vi "Read Oil Presence.vi"(0 "Session Handle in":T1, 11 "error in (no error)":errorcluster) -> (4 "Session Handle out":T1, 6 "Present?":bool, 15 "error out":errorcluster)   [LabVIEW 2015, in "Gas.lvclass"]
uses:
  Gas.lvclass
  Typedefs/Session Handle.ctl
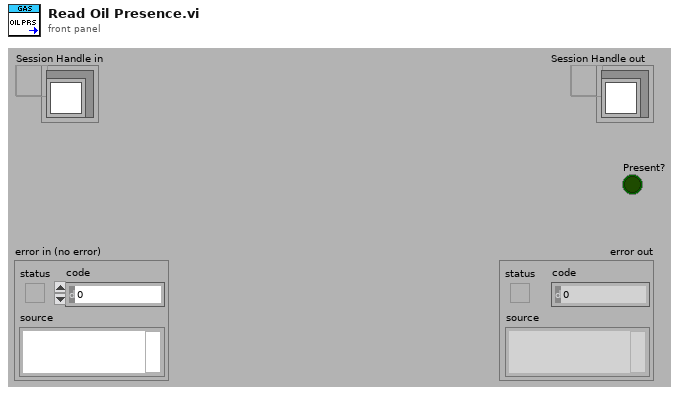
[diagram p1: front panel]
types:
  T1 = typedef "Gas.lvclass/Session Handle.ctl" = refnum<data-value>
  T2 = typedef "XNET Frame CAN.ctl" = cluster{"timestamp":timestamp, "payload":u8[], "identifier":u32, "type":T3, "extended?":bool, "echo?":bool}
  T3 = typedef "XNET Frame Type CAN.ctl" = u8
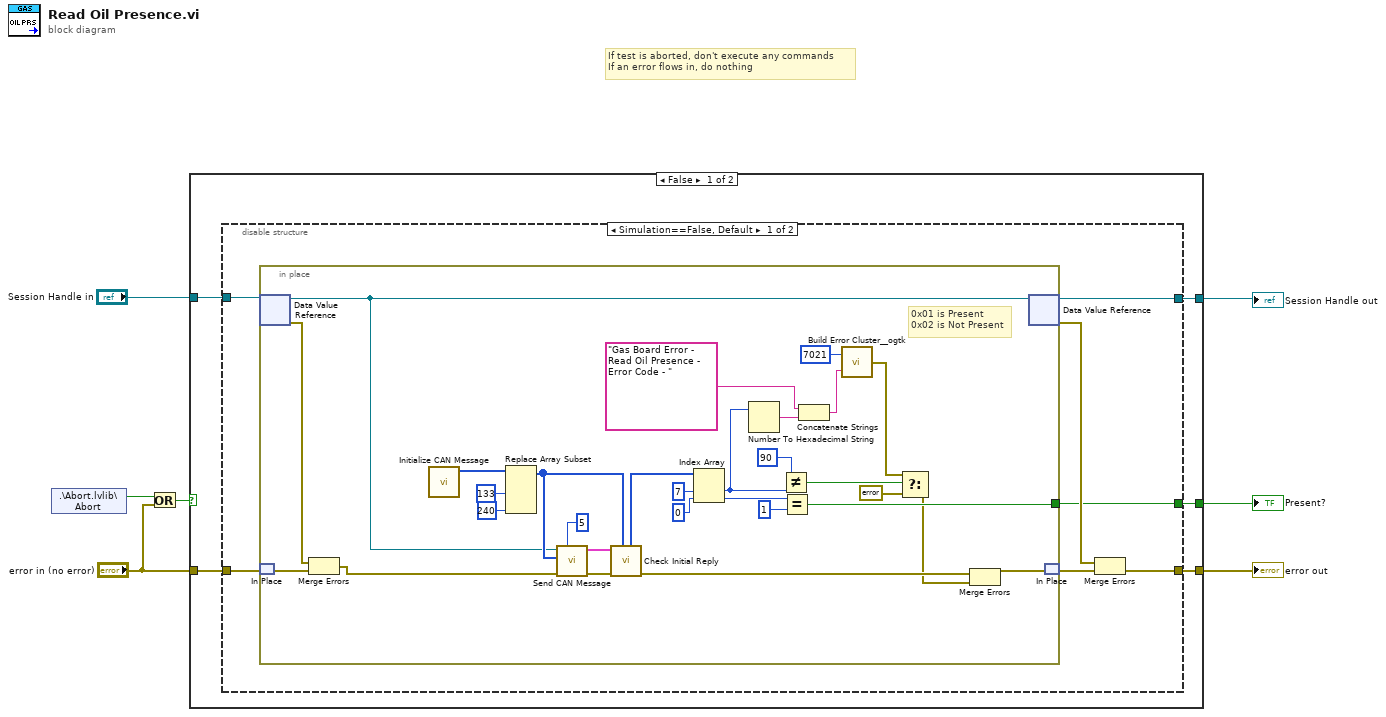
[diagram p0: block diagram]
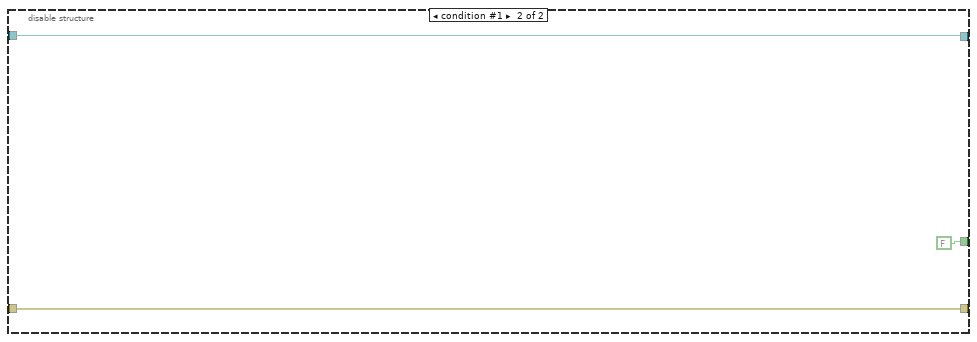
[diagram p2: hidden frame]
diagram:
  # "If test is aborted, don't execute any commands\nIf an error flows in, do nothing"
  n1 = shared-variable ".\\Abort.lvlib\\Abort"() -> (w4:bool)  [unwired: 1 in, 1 out]
  n2 = Or(x=w4, y="error in (no error)") -> (x .or. y?=w2:bool)
  n3 = case shown="False" w2 {
    tunnel: [w12 w53] -> w6
    tunnel: [w11 w52] -> w5
    tunnel: "Session Handle in" -> [w10 w53]
    tunnel: "error in (no error)" -> [w9 w52]
    tunnel: [w8 _] -> w1
    frame False {
      n4 = disable-structure shown="Simulation==False, Default" {
        disable-tunnel: [w19 w51] -> w12
        disable-tunnel: [w16 w50] -> w11
        disable-tunnel: w10 -> [w15 w51]
        disable-tunnel: w9 -> [w14 w50]
        disable-tunnel: [w13 FALSE] -> w8
        frame condition #0 (active) {
          n5 = in-place {
            in-place-border: [w31] -> w13
            # "0x01 is Present\n0x02 is Not Present"
            n6 = in-place-dvr #1(w15) -> (w25:refnum<class "Gas.lvclass">, w44:errorcluster)
            n7 = in-place-match #2(w14) -> (w43:errorcluster)
            n8 = Merge Errors(w44, w43) -> (w24:errorcluster)
            n9 = call "Initialize CAN Message.vi"() -> ("Initial Payload"=w45:u8[])  [unwired: 11 in]
            n10 = Replace Array Subset(array=w45, new element #1=u8 133 ("new element/subarray"), new element #2=u8 240 ("new element/subarray")) -> (w42:u8[])  [unwired: 2 in]
            n11 = call "Send CAN Message.vi"("Number of Retries"=5, "error in (no error)"=w24, "payload"=w42, "Gas In"=w25) -> ("error out"=w22:errorcluster, "Reply"=w40:T2[])  [unwired: 5 in, 1 out]
            n12 = call "Check Initial Reply.vi"("Write Message"=w42, "error in (no error)"=w22, "Reply"=w40) -> ("error out"=w21:errorcluster, "Whole Payload"=w23:u8[])  [unwired: 5 in, 2 out]
            n13 = Index Array(array=w23, index #1=7 ("index"), index #2=0 ("index")) -> (element #1=w30:u8, element #2=w33:u8)
            n14 = Number To Hexadecimal String(2:w30) -> (0:w28:string)  [unwired: 1 in]
            n15 = Not Equal?(x=u8 90 ("new element/subarray"), y=w30) -> (x != y?=w36:bool)
            n16 = Equal?(x=w33, y=u8 1) -> (x = y?=w31:bool)
            n17 = Concatenate Strings("Gas Board Error - Read Oil Presence - Error Code - " ("string"), w28) -> (w26:string)
            n18 = call <userlib>:"Build Error Cluster__ogtk.vi"("String to Prepend to source (\"\")"=w26, "code"=7021) -> ("error out"=w38:errorcluster)
            n19 = Select(t=w38, s=w36, f=errorcluster {"status"=FALSE, "code"=0, "source"=""}) -> (s? t:f=w20:errorcluster)
            n20 = Merge Errors(w21, w20) -> (w46:errorcluster)
            n21 = in-place-dvr #1(w25) -> (w19:T1, w17:errorcluster)
            n22 = in-place-match #2(w46) -> (w18:errorcluster)
          }
          n23 = Merge Errors(w17, w18) -> (w16:errorcluster)
        }
        frame condition #1 {
        }
      }
    }
    frame True {
    }
  }
  "Session Handle out" <- w6
  "error out" <- w5
  "Present?" <- w1
